vi "xwav_limits.vi"(5 "xwave":T1={"attributes"=variant, "X"={"start"=0.0, "delta"=0.0, "units"="index", "dim"="au"}, "Y"={"data"=[], "units"="au"}}) -> (6 "dup xwave":T1={"attributes"=variant, "X"={"start"=0.0, "delta"=0.0, "units"="index", "dim"="au"}, "Y"={"data"=[], "units"="au"}}, 8 "x start":dbl, 10 "x end":dbl)   [LabVIEW 2015]
uses:
  xwav.ctl
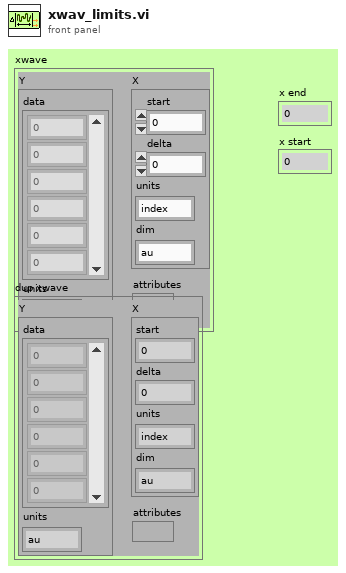
[diagram p1: front panel]
types:
  T1 = typedef "xwav.ctl" = cluster{"attributes":variant, "X":cluster{"start":dbl, "delta":dbl, "units":string, "dim":string}, "Y":cluster{"data":dbl[], "units":string}}
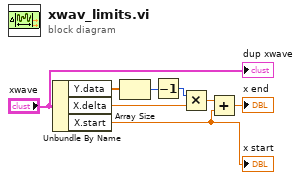
[diagram p0: block diagram]
diagram:
  n1 = Unbundle By Name("xwave") -> ("Y.data"=w8:dbl[], "X.delta"=w5:dbl, "X.start"=w3:dbl)
  "x start" <- w3
  n2 = Array Size(array=w8) -> (size(s)=w7:i32)
  n3 = Decrement(x=w7) -> (x-1=w6:i32)
  n4 = Multiply(x=w6, y=w5) -> (x*y=w2:dbl)
  n5 = Add(x=w2, y=w3) -> (x+y=→"x end":dbl)
  "dup xwave" <- "xwave"
